vi "Grab Tag Information - Decorations.vi"(8 "error in":errorcluster, 11 "VI Ref in":refnum<vi>) -> (0 "error out":errorcluster, 1 "Control Info":T1[](array[typedef]) {"Decoration Level" items=["N/A", "Primary", "Secondary", "Tertiary", "Error", "Primary Fixed", "Secondary Fixed", "Tertiary Fixed", "Label Only", "No Change"]}, 2 "map data":map{string, refnum<vi>}(c390), 3 "VI Ref out":refnum<vi>)   [LabVIEW 2021]
doc: "Get the Tag Data for the decorations on the block diagram (ignores free labels). \n\n<b>Code Developed By:</b>\nDaniel Coons\nTechnology Service Corporation\nwww.tsc.com/atcs"
uses:
  <vilib>/Utility/traverseref.llb/TRef TravTarget.ctl
  <vilib>/Utility/traverseref.llb/VI Scripting - Traverse.lvlib
  Material SubVIs/Material SubVIs.lvlib
  decorations info--typedef.ctl
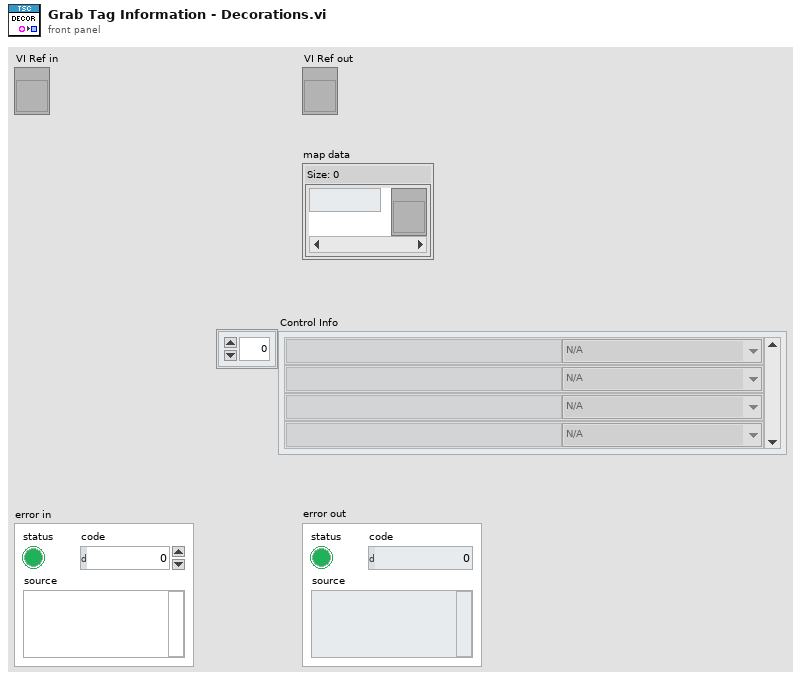
[diagram p1: front panel]
types:
  T1 = typedef "decorations info--typedef.ctl" = cluster{"label":string, "Decoration Level":u16}
  T2 = typedef "TRef TravTarget.ctl" = enum16{"FP", "BD", "Other"}
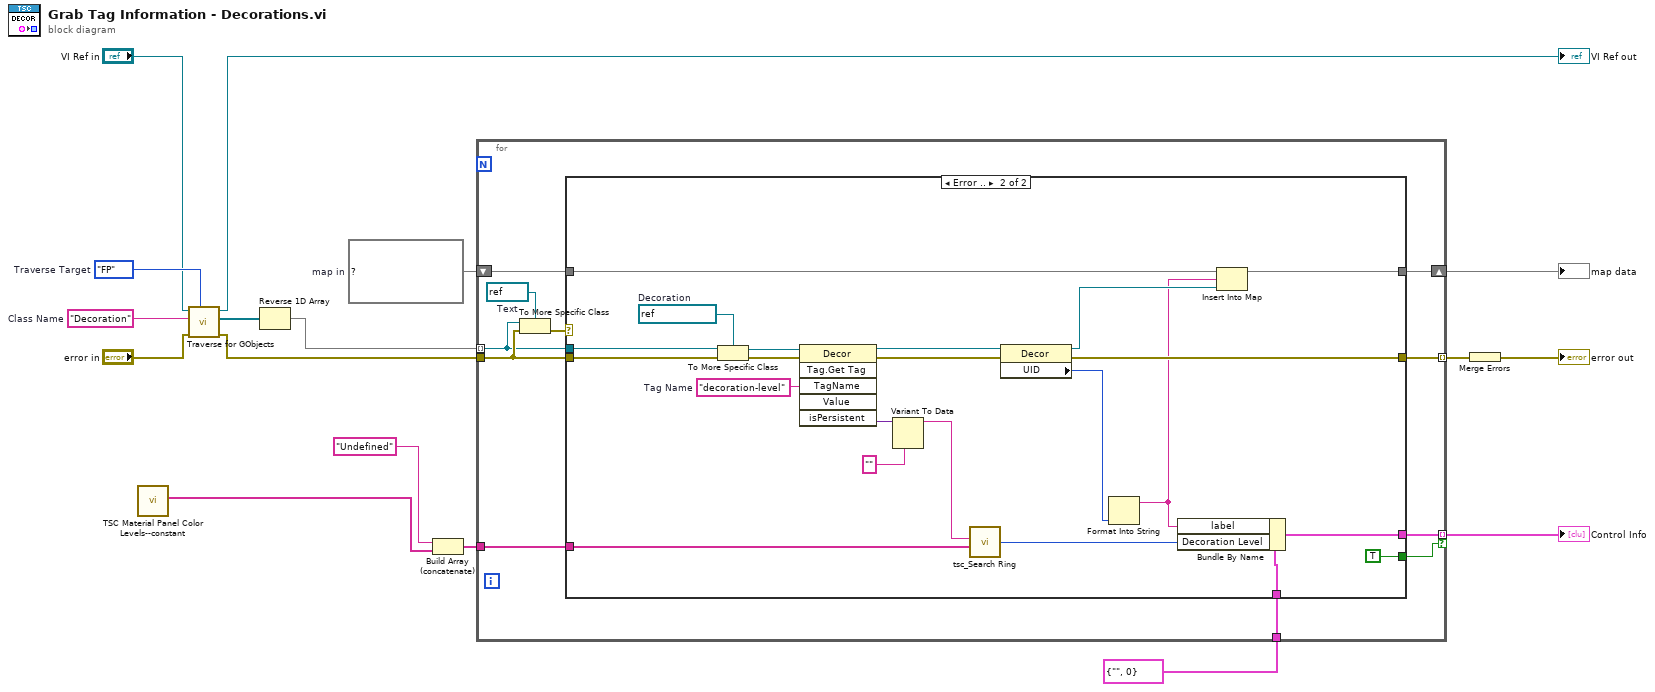
[diagram p0: block diagram]
diagram:
  w9 = TRef_TravTarget."FP"  # Traverse Target
  w10 = "Decoration"  # Class Name
  w14 = map{string, refnum<vi>} {}  # map in
  n1 = call "TSC Material Panel Color Levels--constant.vi"() -> ("front panel color levels"=w2:string[])  [unwired: 11 in]
  n2 = call <vilib>:"Traverse for GObjects.vi"("Traverse Target"=w9, "error in (no error)"="error in", "Class Name"=w10, "VI Refnum"="VI Ref in") -> ("error out"=w16:errorcluster, "References"=w8:refnum<vi>[], "dup VI Refnum"=→"VI Ref out":refnum<vi>)  [unwired: 4 in, 1 out]
  n3 = Reverse 1D Array(array=w8) -> (reversed array=w6:refnum<vi>[])
  n4 = Build Array (concatenate)("Undefined", w2) -> (w11:string[])
  n5 = for {
    tunnel: w6 -> [w21] mode=indexing
    tunnel: w16 -> [w22]
    tunnel: [w28] -> w5 mode=indexing
    tunnel: T1 {"label"="", "Decoration Level"=0} ("decoration info") -> [w27]
    tunnel: [w26] -> w13 mode=indexing if=w18
    shift-right: [w24] -> w1
    shift-left: w14 -> [w25]
    tunnel: w11 -> [w23]
    w19 = refnum<vi> refnum  # Text
    n6 = To More Specific Class(target class=w19, reference=w21, error in=w22) -> (error out=w20:errorcluster)  [unwired: 1 out]
    n7 = case shown="Error .." w20 {
      tunnel: w22 -> [w29 w52]
      tunnel: [w29 w50] -> w28
      tunnel: w27 -> [_ w43]
      tunnel: [_ w42] -> w26
      tunnel: w25 -> [w30 w41]
      tunnel: [w30 w40] -> w24
      tunnel: w23 -> [_ w39]
      tunnel: w21 -> [_ w38]
      tunnel: [_ TRUE] -> w18
      frame No Error {
      }
      frame Error {
        w44 = refnum<vi> refnum  # Decoration
        w48 = "decoration-level"  # Tag Name
        n8 = To More Specific Class(target class=w44, reference=w38, error in=w52) -> (specific class reference=w45:refnum<vi>, error out=w49:errorcluster)
        n9 = invoke class="Decor" method="Tag.Get Tag"(reference=w45, error in=w49, "TagName"=w48) -> (reference out=w37:refnum<vi>, error out=w51:errorcluster, "isPersistent"=w47:variant)  [unwired: 3 in, 3 out]
        n10 = Variant To Data(type="", Variant=w47) -> (data=w36:string)  [unwired: 1 in, 1 out]
        n11 = call "tsc_Search Ring.vi"("Values"=w39, "Search Item"=w36) -> ("Index"=w35:u16)  [unwired: 2 in]
        n12 = property class="Decor"(reference=w37, error in=w51) -> (reference out=w33:refnum<vi>, error out=w50:errorcluster, "UID"=w34:i32)
        n13 = Format Into String(w34) -> (resulting string=w32:string)  [unwired: 3 in, 1 out]
        n14 = Bundle By Name(cluster=w43, "label"=w32, "Decoration Level"=w35) -> (w42:T1)
        n15 = Insert Into Map(map in=w41, key=w32, value=w33) -> (map out=w40:map{string, refnum<vi>})  [unwired: 2 out]
      }
    }
  }
  "Control Info" <- w13
  "map data" <- w1
  n16 = Merge Errors(w5) -> (→"error out":errorcluster)
